vi "get channel group.vi"(8 "error in":errorcluster, 10 "channel classification":T2, 11 "channels":refnum<class "TBM channel.lvclass">[](array[class])) -> (0 "error out":errorcluster, 2 "data table":T1, 3 "dictionary":refnum<class "data dictionary.lvclass">)   [LabVIEW 2013, in "TBM channel.lvclass"]
doc: "Filters a list of channels by classification and returns the tag bus and data table associated with this classification."
uses:
  TBM channel.lvclass
  channel classification.ctl
  <vilib>/NI/Tag Bus/table/data table.ctl
  <vilib>/NI/Tag Bus/dictionary/data dictionary.lvclass
  TBM channel.lvclass/TBM channel.ctl
  <vilib>/NI/Tag Bus/dictionary/data dictionary.lvclass/data dictionary.ctl
  <vilib>/NI/Tag Bus/table/data table.lvlib
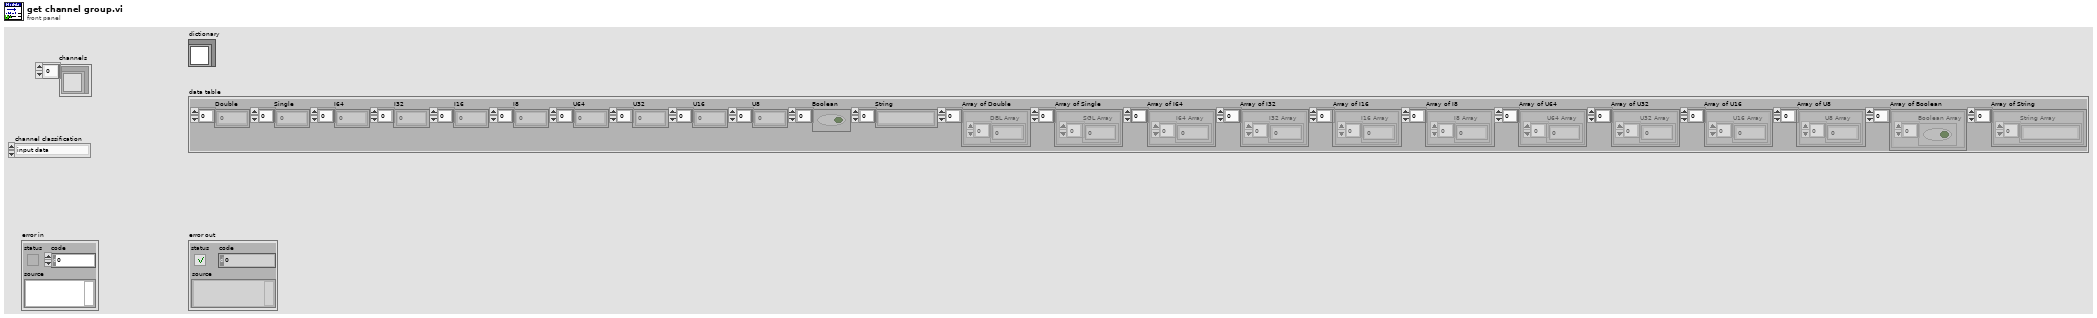
[diagram p1: front panel]
types:
  T1 = typedef "tag bus.lvlib/data table.lvlib/data table.ctl" = cluster{"Double":dbl[], "Single":sgl[], "I64":i64[], "I32":i32[], "I16":i16[], "I8":i8[], "U64":u64[], "U32":u32[], "U16":u16[], "U8":u8[], "Boolean":bool[], "String":string[], "Array of Double":cluster{"DBL Array":dbl[]}[], "Array of Single":cluster{"SGL Array":sgl[]}[], "Array of I64":cluster{"I64 Array":i64[]}[], "Array of I32":cluster{"I32 Array":i32[]}[], "Array of I16":cluster{"I16 Array":i16[]}[], "Array of I8":cluster{"I8 Array":i8[]}[], "Array of U64":cluster{"U64 Array":u64[]}[], "Array of U32":cluster{"U32 Array":u32[]}[], "Array of U16":cluster{"U16 Array":u16[]}[], "Array of U8":cluster{"U8 Array":u8[]}[], "Array of Boolean":cluster{"Boolean Array":bool[]}[], "Array of String":cluster{"String Array":string[]}[]}
  T2 = typedef "TBM channel.lvclass/channel classification.ctl" = enum16{"input data", "output data", "processing parameter", "processing result"}
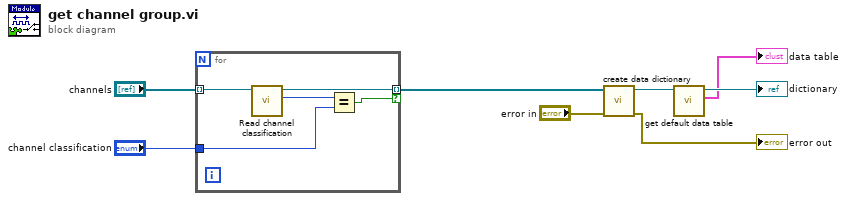
[diagram p0: block diagram]
diagram:
  n1 = for {
    tunnel: "channels" -> [w12] mode=indexing
    tunnel: "channel classification" -> [w13]
    tunnel: [w10] -> w3 mode=indexing if=w9
    n2 = call "Read channel classification.vi"("channel in"=w12) -> ("channel classification"=w11:T2, "channel out"=w10:refnum<class "TBM channel.lvclass">)  [unwired: 8 in, 1 out]
    n3 = Equal?(x=w11, y=w13) -> (x = y?=w9:bool)
  }
  n4 = call <vilib>:"create data dictionary.vi"("error in"="error in", "system tags"=w3) -> ("error out"=→"error out":errorcluster, "data dictionary"=w4:refnum<class "data dictionary.lvclass">)  [unwired: 8 in]
  n5 = call <vilib>:"get default data table.vi"("data dictionary in"=w4) -> ("default data table"=→"data table":T1, "data dictionary out"=→"dictionary":refnum<class "data dictionary.lvclass">)  [unwired: 9 in]
